vi "Read inputs.vi"(9 "Node in":refnum<class "Node.lvclass">) -> (3 "Node out":refnum<class "Node.lvclass">, 4 "inputs":refnum<class "Terminal.lvclass">[](array[class]))   [LabVIEW 2014, in "Node.lvclass"]
uses:
  Node.lvclass
  Terminal/Terminal.lvclass
  Node.lvclass/Node.ctl
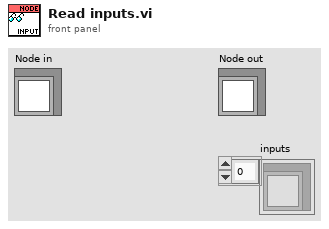
[diagram p1: front panel]
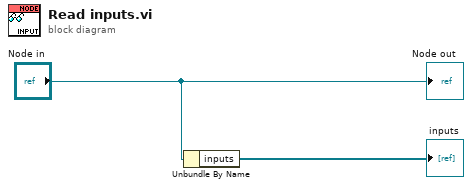
[diagram p0: block diagram]
diagram:
  n1 = Unbundle By Name("Node in") -> ("inputs"=→"inputs":refnum<class "Terminal.lvclass">[])
  "Node out" <- "Node in"
